vi "Alias.vi"(11 "Alias":string) -> (3 "Data":string)   [LabVIEW 2020]
uses:
  <vilib>/Utility/config.llb/Read Key (String).vi
  <vilib>/Utility/config.llb/NI_LVConfig.lvlib
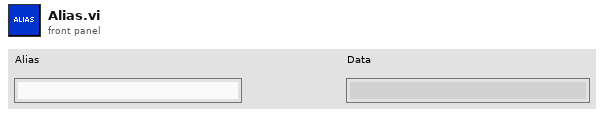
[diagram p1: front panel]
types:
  T1 = typedef "NI_LVConfig.lvlib/Config Data RefNum.ctl" = refnum<k1>
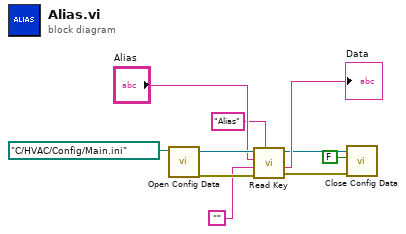
[diagram p0: block diagram]
diagram:
  n1 = call <vilib>:"Open Config Data.vi"("configuration file path"=path "C:/HVAC/Config/Main.ini") -> ("error out"=w9:errorcluster, "refnum"=w8:T1)  [unwired: 8 in, 1 out]
  n2 = call-poly <vilib>:"Read Key.vi"("section"="Alias", "error in (no error)"=w9, "default value"="", "key"="Alias", "refnum"=w8) -> ("error out"=w3:errorcluster, "value"=→"Data":string, "refnum out"=w2:T1)  [unwired: 3 in, 1 out]
  n3 = call <vilib>:"Close Config Data.vi"("error in (no error)"=w3, "write file if changed (T)"=FALSE, "refnum"=w2) -> ()  [unwired: 7 in, 2 out]
